vi "wGetWl.vi"(3 "error in (no error)":errorcluster, 5 "SpectRef In":T1) -> (0 "error out":errorcluster, 1 "WL Values":dbl[](array[numeric]), 2 "SpectRef Out":T1)   [LabVIEW 2012]
uses:
  Controls/USB4000_Data.ctl
panel:
  out "appended path 2":path
  out "appended path":path
  out "Length":i32
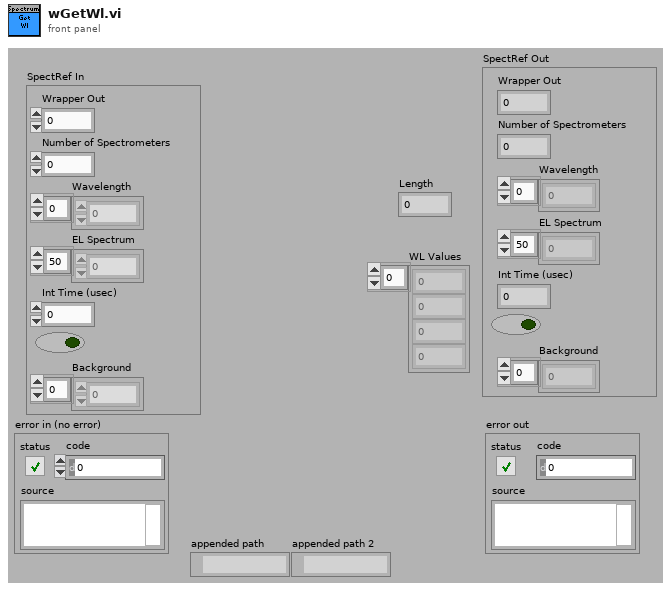
[diagram p1: front panel]
types:
  T1 = typedef "USB4000_Data.ctl" = cluster{"Wrapper Out":u32, "Number of Spectrometers":i32, "Wavelength":dbl[], "EL Spectrum":dbl[], "Int Time (usec)":i32, bool, "Background":dbl[]}
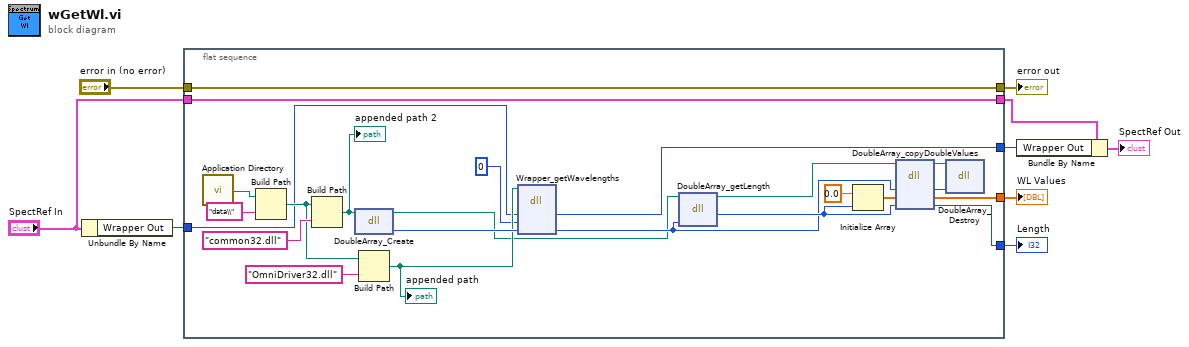
[diagram p0: block diagram]
diagram:
  n1 = Unbundle By Name("SpectRef In") -> ("Wrapper Out"=w5:u32)
  n2 = flat-sequence {
    tunnel: [w27] -> w9
    tunnel: [w26] -> w8
    tunnel: [w14] -> w7
    tunnel: "error in (no error)" -> [w14]
    tunnel: w5 -> [w12]
    tunnel: "SpectRef In" -> [w11]
    tunnel: [w11] -> w2
    tunnel: [w10] -> w1
    frame #0 {
      n3 = call <vilib>:"Application Directory.vi"() -> ("Application Directory"=w24:path)
      n4 = Build Path(base path=w24, name or relative path="data\\") -> (appended path=w19:path)
      n5 = Build Path(base path=w19, name or relative path="common32.dll") -> (appended path=w15:path)
      "appended path 2" <- w15
      n6 = dll-call lib="common32.dll" fn="DoubleArray_Create" label="DoubleArray.Create"(path in=w15) -> (path out=w18:path, "return type"=w32:u32)  [unwired: 2 in, 1 out]
      n7 = Build Path(base path=w19, name or relative path="OmniDriver32.dll") -> (appended path=w20:path)
      "appended path" <- w20
      n8 = dll-call lib="D:/Software Development/EPI Development/BurnIn Testing/Instruments/Drivers/Ocean Optics/OOI_HOME/OmniDriver32.dll" fn="Wrapper_getWavelengths" label="Wrapper.getWavelengths"(path in=w20, "Wrapper"=w12, "Index"=0, "WL DoubleArray"=w32) -> ("Wrapper"=w10:u32, "WL DoubleArray"=w28:u32)  [unwired: 3 in, 3 out]
      n9 = dll-call lib="common32.dll" fn="DoubleArray_getLength" label="DoubleArray.getLength"(path in=w18, "DoubbleArray"=w28) -> (path out=w17:path, "return type"=w30:i32)  [unwired: 3 in, 1 out]
      n10 = Initialize Array(0.0 ("element"), w30) -> (w29:dbl[])
      n11 = dll-call lib="common32.dll" fn="DoubleArray_copyDoubleValues" ("DoubleArray.coopyDoubleValues")(path in=w17, "DoubleArray"=w28, "Values"=w29, "Length"=w30) -> (path out=w16:path, "DoubleArray"=w25:u32, "Values"=w27:dbl[], "Length"=w26:i32)  [unwired: 2 in, 2 out]
      n12 = dll-call lib="common32.dll" fn="DoubleArray_Destroy" ("DoubleArray.Destroy")(path in=w16, "DoubleArray"=w25) -> ()  [unwired: 3 in, 3 out]
    }
  }
  n13 = Bundle By Name(cluster=w2, "Wrapper Out"=w1) -> (→"SpectRef Out":T1)
  "WL Values" <- w9
  "Length" <- w8
  "error out" <- w7
